vi "MongoDB.CollectionDropAll.vi"(8 "error in (no error)":errorcluster, 11 "MongoDB.Collection in":refnum<class "MongoDB.Collection.lvclass">) -> (0 "error out":errorcluster, 3 "MongoDB.Collection out":refnum<class "MongoDB.Collection.lvclass">)   [LabVIEW 2014, in "MongoDB.Collection.lvclass"]
uses:
  MongoDB.Collection.lvclass
  MongoDB.Collection.lvclass/MongoDB.Collection.ctl
  C:/MongoData/Drivers/mongo-csharp-driver-2.0.0-beta4/mongo-csharp-driver-2.0.0-beta4/src/MongoDB.Driver.Legacy/bin/Release/MongoDB.Driver.Legacy.dll
  MongoData/Drivers/mongo-csharp-driver-2.0.0-beta4/mongo-csharp-driver-2.0.0-beta4/src/MongoDB.Driver.Legacy/bin/Release/MongoDB.Driver.Legacy.dll
  MongoDB.Database.lvclass
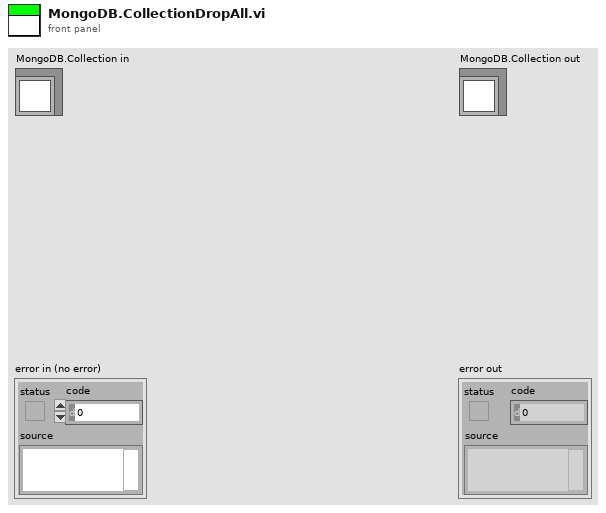
[diagram p1: front panel]
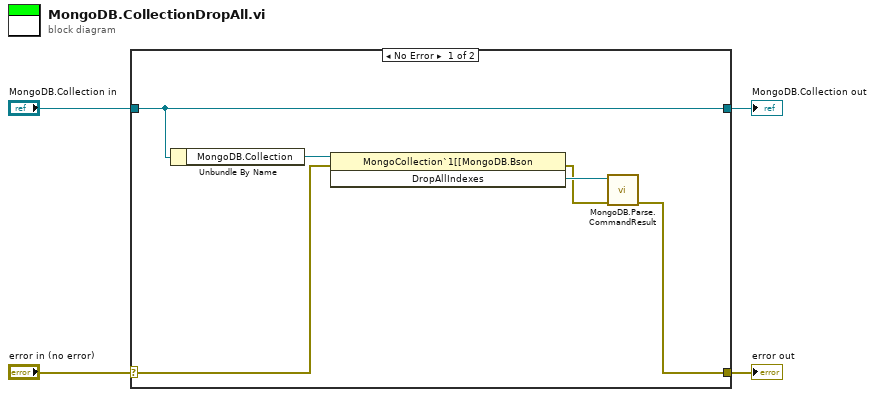
[diagram p0: block diagram]
diagram:
  n1 = case shown="No Error" "error in (no error)" {
    selector: "error in (no error)" -> [w5 w12]
    tunnel: [w6 w12] -> w3
    tunnel: [w10 w11] -> w1
    tunnel: "MongoDB.Collection in" -> [w10 w11]
    frame No Error {
      n2 = Unbundle By Name(w10) -> ("MongoDB.Collection"=w9:refnum<k24>)
      n3 = invoke class="MongoCollection`1[[MongoDB.Bson" method="DropAllIndexes"(reference=w9, error in=w5) -> (error out=w7:errorcluster, "DropAllIndexes"=w8:refnum<k24>)  [unwired: 1 in, 1 out]
      n4 = call "MongoDB.Parse.CommandResult.vi"("error in (no error)"=w7, "MongoDB.Command.Result"=w8) -> ("error out"=w6:errorcluster)  [unwired: 9 in]
    }
    frame Error {
    }
  }
  "error out" <- w3
  "MongoDB.Collection out" <- w1
